vi "Uv1_2022.vi"(1 "Temperature [K]":dbl format="%.4f", 2 "xw":dbl, 3 "Gamma0 humid air":dbl) -> (0 "Uv1":dbl)   [LabVIEW 2016]
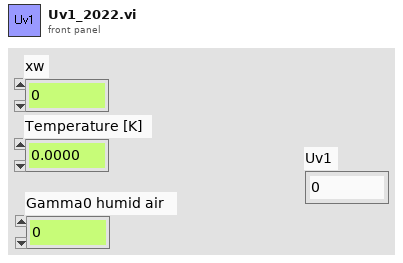
[diagram p1: front panel]
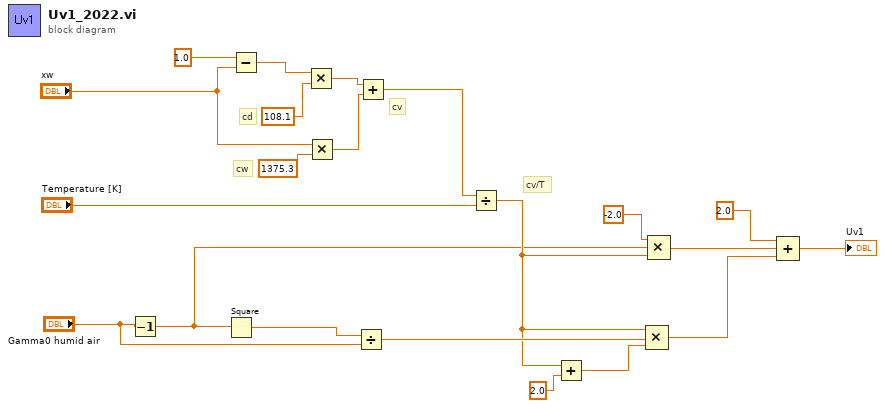
[diagram p0: block diagram]
diagram:
  # "cv/T"
  # "cv"
  # "cw"
  # "cd"
  n1 = Decrement(x="Gamma0 humid air") -> (x-1=w1:dbl)
  n2 = Square(x=w1) -> (x^2=w11:dbl)
  n3 = Subtract(x=1.0, y="xw") -> (x-y=w19:dbl)
  n4 = Multiply(x=w19, y=108.1) -> (x*y=w17:dbl)
  n5 = Multiply(x="xw", y=1375.3) -> (x*y=w14:dbl)
  n6 = Divide(x=w11, y="Gamma0 humid air") -> (x/y=w10:dbl)
  n7 = Add(x=w17, y=w14) -> (x+y=w13:dbl)
  n8 = Divide(x=w13, y="Temperature [K]") -> (x/y=w9:dbl)
  n9 = Add(x=w9, y=2.0) -> (x+y=w7:dbl)
  n10 = Compound Arithmetic op=MULTIPLY(w9, w10, w7) -> (w5:dbl)
  n11 = Compound Arithmetic op=MULTIPLY(-2.0 ("value"), w1, w9) -> (w3:dbl)
  n12 = Compound Arithmetic op=ADD(2.0 ("x"), w3, w5) -> (→"Uv1":dbl)
